vi "InitResultFile.vi"(8 "error in (no error)":errorcluster, 11 "PmuDelayClass in":refnum<class "PmuDelay.lvclass">) -> (0 "error out":errorcluster, 3 "PmuDelayClass out":refnum<class "PmuDelay.lvclass">)   [LabVIEW 2018, in "AnalysisPlugins.lvlib" / "PmuDelay.lvclass"]
uses:
  PmuDelay.lvclass
  C:/projects/ICDAS/NistPluggableModules/Analysis/AnalysisPlugins/AnalysisPluginBaseClass/AnalysisPluginsBase.lvclass
  FGen/MemberClasses/PmuTestFunctions/Typedefs/PmuTestParams.ctl
  AnalysisPluginBaseClass/AnalysisPluginsBase.lvclass/AnalysisPluginsBase.ctl
  AnalysisPluginBaseClass/Accessors/Read ResultPath.vi
  AnalysisPluginBaseClass/Accessors/Read FileName.vi
  <vilib>/Utility/file.llb/Write Delimited Spreadsheet (string).vi
  FGen/MemberClasses/PmuTestFunctions/PmuTestFunctions.lvclass
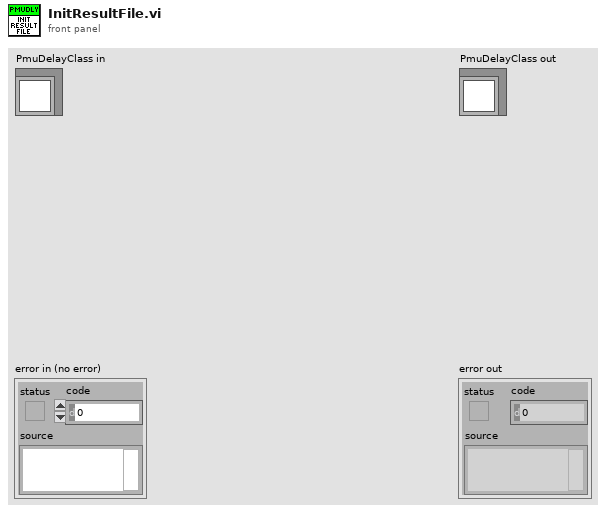
[diagram p1: front panel]
types:
  T1 = typedef "Functions.lvlib/PmuTestFunctions.lvclass/PmuTestParams.ctl" = dbl[][]
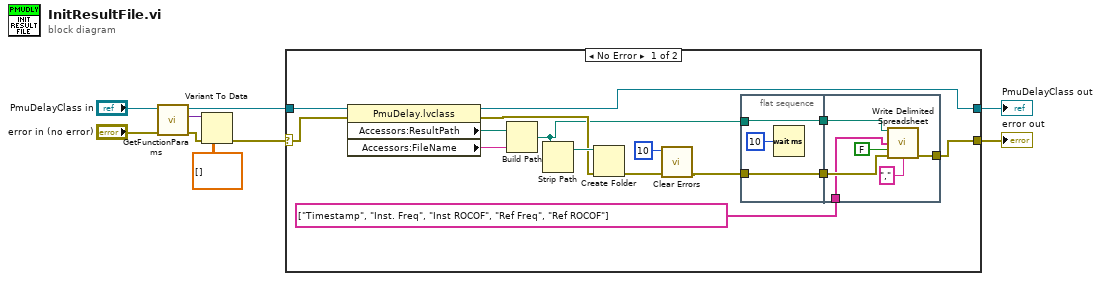
[diagram p0: block diagram]
diagram:
  n1 = call-dynamic "GetFunctionParams.vi"("error in (no error)"="error in (no error)", "PmuAnalysis in"="PmuDelayClass in") -> ("error out"=w2:errorcluster, "FunctionParams"=w4:variant, "PmuAnalysis out"=w6:refnum<class "PmuDelay.lvclass">)  [unwired: 7 in]
  n2 = Variant To Data(error in=w2, type=T1 [] ("Accessors:PmuTestParams"), Variant=w4) -> (error out=w1:errorcluster)  [unwired: 1 out]
  n3 = case shown="No Error" w1 {
    selector: w1 -> [w10 w34]
    tunnel: [w11 w34] -> w9
    tunnel: [w12 w35] -> w8
    tunnel: w6 -> [w24 w35]
    frame No Error {
      n4 = property class="PmuDelay.lvclass"(reference=w24, error in=w10) -> (reference out=w12:refnum<class "PmuDelay.lvclass">, error out=w20:errorcluster, "Accessors:ResultPath"=w23:path, "Accessors:FileName"=w22:string)
      n5 = Build Path(base path=w23, name or relative path=w22) -> (appended path=w14:path)
      n6 = Strip Path(path=w14) -> (stripped path=w21:path)  [unwired: 1 out]
      n7 = Create Folder(path (use dialog)=w21, error in=w20) -> (error out=w18:errorcluster)  [unwired: 1 in, 2 out]
      n8 = call <vilib>:"Clear Errors.vi"("error in (no error)"=w18, "specific error code to clear (0: all)"=10) -> ("error out"=w17:errorcluster)  [unwired: 4 in, 1 out]
      n9 = flat-sequence {
        tunnel: w17 -> [w26]
        tunnel: [w26] -> w16
        tunnel: w14 -> [w25]
        tunnel: [w25] -> w15
        tunnel: w16 -> [w32]
        tunnel: w15 -> [w30]
        tunnel: string[] ["Timestamp", "Inst. Freq", "Inst ROCOF", "Ref Freq", "Ref ROCOF"] -> [w29]
        tunnel: [w28] -> w11
        frame #0 {
          n10 = Wait (ms)(milliseconds to wait=u32 10) -> ()  [unwired: 1 out]
        }
        frame #1 {
          n11 = call-poly <vilib>:"Write Delimited Spreadsheet.vi"("file path (dialog if empty)"=w30, "1D data"=w29, "append to file? (new file:F)"=FALSE, "error in (no error)"=w32, "delimiter (\\t)"="," ("delimiter (\\t)")) -> ("error out"=w28:errorcluster)  [unwired: 9 in, 1 out]
        }
      }
    }
    frame Error {
    }
  }
  "error out" <- w9
  "PmuDelayClass out" <- w8
